vi "751MainControl_Hardware.vi"() -> ()   [LabVIEW 2026]
panel:
  out "Motor State":string
  out "Controller Output Chart":dbl(graph)
  out "Target Resistance Chart":dbl(graph)
  out "Measured Resistance Chart":dbl(graph)
  out "Controller Output":dbl
  out "Error":dbl
  out "Target Resistance":dbl
  out "Measured Resistance":dbl
  in  "Kc":dbl
  in  "Bound":dbl
  in  "stop":bool
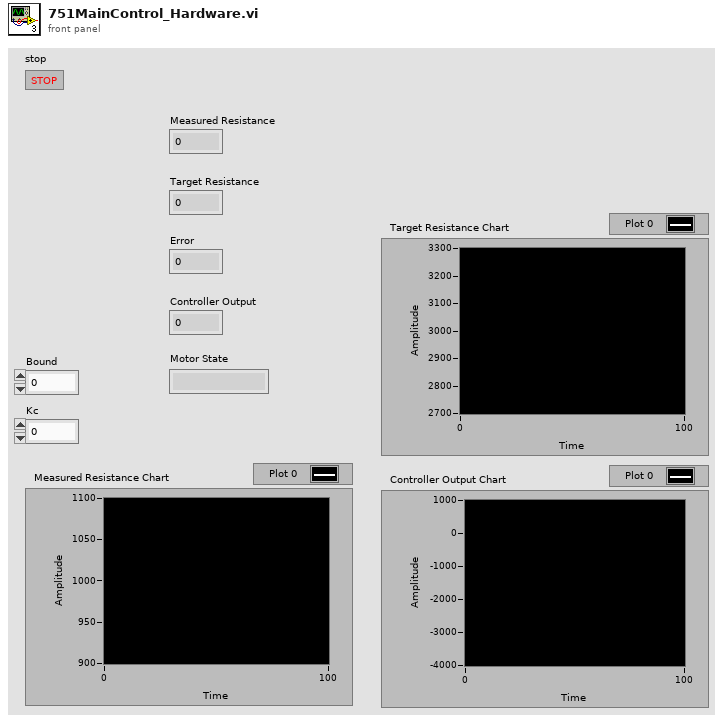
[diagram p1: front panel]
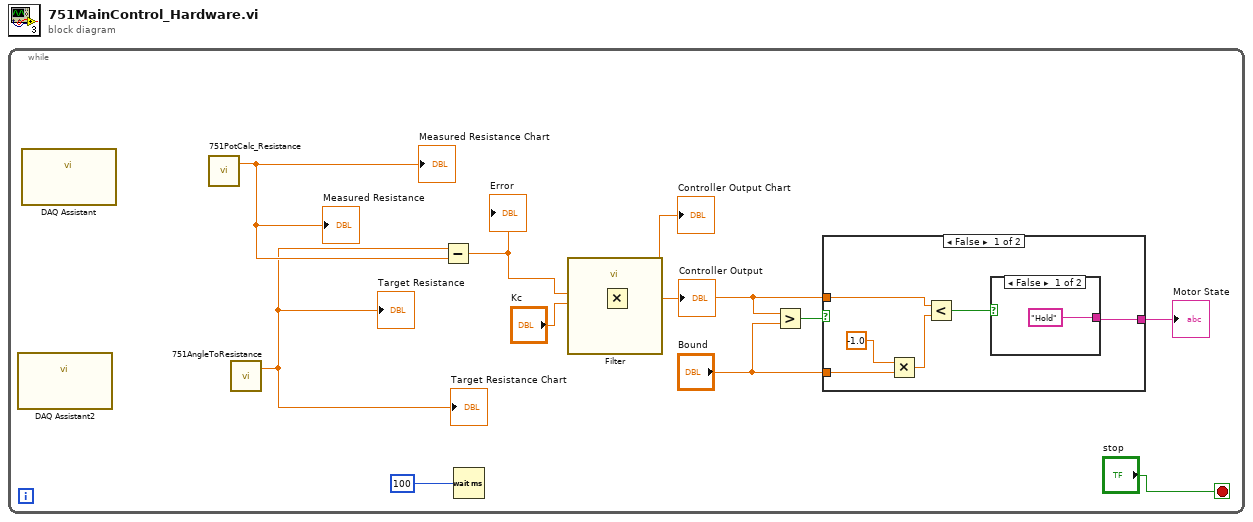
[diagram p0: block diagram]
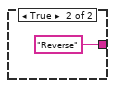
[diagram p2: hidden frame]
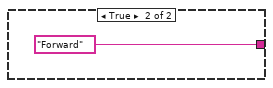
[diagram p3: hidden frame]
diagram:
  n1 = while {
    stop <- "stop" stop-if-true
    n2 = call "DAQ Assistant2"() -> ()  [unwired: 12 in]
    n3 = call "DAQ Assistant"() -> ()  [unwired: 12 in]
    n4 = call "751PotCalc_Resistance.vi"() -> ("Vout"=w12:dbl, "Rx"=w6:dbl, "Vin"=w13:dbl, "R1"=w14:dbl)
    "Measured Resistance" <- w6
    "Measured Resistance Chart" <- w6
    n5 = call "751AngleToResistance.vi"() -> ("180 deg resistance"=w9:dbl, "Resistance"=w5:dbl, "0 deg resistance"=w11:dbl, "Angle"=w10:dbl)
    "Target Resistance" <- w5
    "Target Resistance Chart" <- w5
    n6 = Subtract(x=w5, y=w6) -> (x-y=w8:dbl)
    "Error" <- w8
    n7 = Wait (ms)(milliseconds to wait=100) -> ()  [unwired: 1 out]
    n8 = Multiply(x=w8, y="Kc") -> (x*y=w3:dbl)
    "Controller Output" <- w3
    "Controller Output Chart" <- w3
    n9 = Greater?(x=w3, y="Bound") -> (0:w2:bool)
    n10 = case shown="False" w2 {
      tunnel: [w17 "Forward"] -> w1
      tunnel: "Bound" -> [w21 _]
      tunnel: w3 -> [w20 _]
      frame False {
        n11 = Multiply(x=-1.0, y=w21) -> (x*y=w19:dbl)
        n12 = Less?(x=w20, y=w19) -> (x < y?=w18:bool)
        n13 = case shown="False" w18 {
          tunnel: ["Hold" "Reverse"] -> w17
          frame False {
          }
          frame True {
          }
        }
      }
      frame True {
      }
    }
    "Motor State" <- w1
  }
  n14 = call "Filter"() -> ()  [unwired: 10 in, 2 out]
